vi "ConvertMac2UnixFiles.vi"(8 "Error In":errorcluster, 11 "Filename":path) -> (0 "Error Out":errorcluster)   [LabVIEW 2010]
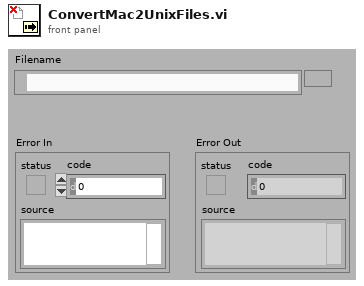
[diagram p1: front panel]
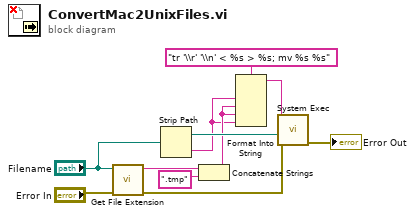
[diagram p0: block diagram]
diagram:
  n1 = call <vilib>:"Get File Extension.vi"("error in (no error)"="Error In", "file"="Filename") -> ("error out"=w4:errorcluster, "filename without extension"=w10:string)  [unwired: 6 in, 2 out]
  n2 = Strip Path(path="Filename") -> (stripped path=w7:path, name=w1:string)
  n3 = Concatenate Strings(w10, ".tmp" ("string")) -> (w2:string)
  n4 = Format Into String(format string="tr '\\r' '\\n' < %s > %s; mv %s %s" ("command line"), w1, w2, w2, w1) -> (resulting string=w5:string)  [unwired: 2 in, 1 out]
  n5 = call <vilib>:"System Exec.vi"("error in (no error)"=w4, "working directory"=w7, "command line"=w5) -> ("error out"=→"Error Out":errorcluster)  [unwired: 5 in, 3 out]
